vi "rvc Rotation Matrix to Euler.vi"(10 "rotation order":T1=11 items=["X-Y-Z", "X-Z-Y", "Y-X-Z", "Y-Z-X", "Z-X-Y", "Z-Y-X", "X-Y-X", "X-Z-X", "Y-X-Y", "Y-Z-Y", "Z-X-Z", "Z-Y-Z"], 11 "rotation matrix":T2) -> (0 "error":i32, 3 "euler angles":cluster{"phi":dbl, "theta":dbl, "psi":dbl})   [LabVIEW 2013]
uses:
  <vilib>/Analysis/Matrix/Datatypes/RealMatrix.ctl
  <vilib>/Analysis/coordinate.llb/Euler Rotation Order.ctl
  <vilib>/Analysis/NI_AALPro.lvlib
  <vilib>/Analysis/Matrix/NI_Matrix.lvlib
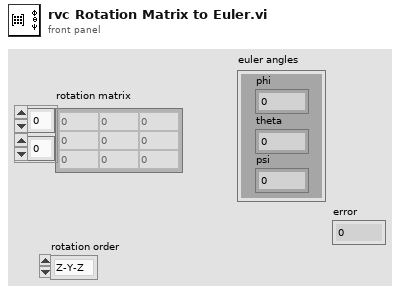
[diagram p1: front panel]
types:
  T1 = typedef "NI_AALPro.lvlib/Euler Rotation Order.ctl" = u16
  T2 = typedef "NI_Matrix.lvlib/RealMatrix.ctl" = dbl[][]
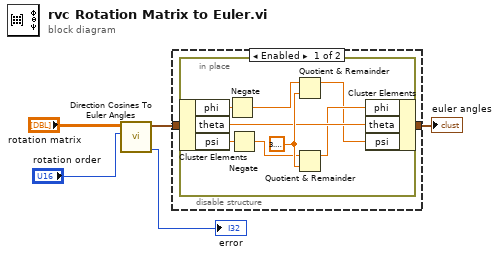
[diagram p0: block diagram]
diagram:
  n1 = call <vilib>:"Direction Cosines To Euler Angles.vi"("rotation order"="rotation order", "Direction Cosines"="rotation matrix") -> ("error"=→"error":i32, "Euler Angles"=w1:cluster{"phi":dbl, "theta":dbl, "psi":dbl})  [unwired: 8 in]
  n2 = disable-structure shown="Enabled" {
    disable-tunnel: [w7 w16] -> w2
    disable-tunnel: w1 -> [w6 w16]
    frame Enabled {
      n3 = in-place {
        w15 = 3.141592653589793
        n4 = in-place-cluster #1(w6) -> ("phi"=w14:dbl, "theta"=w13:dbl, "psi"=w12:dbl)
        n5 = Negate(x=w14) -> (-x=w9:dbl)
        n6 = Negate(x=w12) -> (-x=w11:dbl)
        n7 = Quotient & Remainder(x=w9, y=w15) -> (x-y*floor(x/y)=w8:dbl)  [unwired: 1 out]
        n8 = Quotient & Remainder(x=w11, y=w15) -> (x-y*floor(x/y)=w10:dbl)  [unwired: 1 out]
        n9 = in-place-cluster #1("phi"=w10, "theta"=w13, "psi"=w8) -> (w7:cluster{"phi":dbl, "theta":dbl, "psi":dbl})
      }
    }
    frame Disabled {
    }
  }
  "euler angles" <- w2
